vi "Y_N_KeyPress.vi"(8 "error in (no error)":errorcluster) -> (0 "error out":errorcluster, 1 "P/F":bool, 2 "PASS/FAIL":string="FAIL", 3 "Y/N":string="No", 4 "numberKey":i32, 5 "keys pressed":T1(array[ring]))   [LabVIEW 2018]
uses:
  <vilib>/Utility/inputDevices.llb/keyboardAcquire.vi
  <vilib>/Utility/inputDevices.llb/closeKeyboard.vi
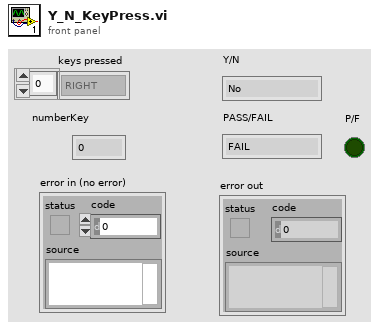
[diagram p1: front panel]
types:
  T1 = enum16{"0", "1", "2", "3", "4", "5", "6", "7", "8", "9", "A", "B", "C", "D", "E", "F", "G", "H", "I", "J", "K", "L", "M", "N", "O", "P", "Q", "R", "S", "T", "U", "V", "W", "X", "Y", "Z", "F1", "F2", "F3", "F4", "F5", "F6", "F7", "F8", "F9", "F10", "F11", "F12", "F13", "F14", "F15", "ADD", "BACK", "BACKSLASH", "CAPITAL", "COMMA", "DECIMAL", "DELETE", "DIVIDE", "DOWN", "END", "EQUALS", "ESCAPE", "GRAVE (`)", "HOME", "INSERT", "LBRACKET", "LCONTROL", "LEFT", "L ALT", "LSHIFT", "LWIN", "MINUS", "MULTIPLY", "NEXT", "NUMLOCK", "NUMPAD_0", "NUMPAD_1", "NUMPAD_2", "NUMPAD_3", "NUMPAD_4", "NUMPAD_5", "NUMPAD_6", "NUMPAD_7", "NUMPAD_8", "NUMPAD_9", "PAUSE", "PERIOD", "PRIOR (PG UP)", "RBRACKET", "RCONTROL", "RETURN", "RIGHT", "R ALT", "RSHIFT", "RWIN", "SCROLL", "SEMICOLON", "SLASH", "SPACE", "SUBTRACT", "TAB", "UP", "ENTER (num pad)", "' (quote)"}[]
  T2 = enum16{"0", "1", "2", "3", "4", "5", "6", "7", "8", "9", "A", "B", "C", "D", "E", "F", "G", "H", "I", "J", "K", "L", "M", "N", "O", "P", "Q", "R", "S", "T", "U", "V", "W", "X", "Y", "Z", "F1", "F2", "F3", "F4", "F5", "F6", "F7", "F8", "F9", "F10", "F11", "F12", "F13", "F14", "F15", "ADD", "BACK", "BACKSLASH", "CAPITAL", "COMMA", "DECIMAL", "DELETE", "DIVIDE", "DOWN", "END", "EQUALS", "ESCAPE", "GRAVE (`)", "HOME", "INSERT", "LBRACKET", "LCONTROL", "LEFT", "L ALT", "LSHIFT", "LWIN", "MINUS", "MULTIPLY", "NEXT", "NUMLOCK", "NUMPAD_0", "NUMPAD_1", "NUMPAD_2", "NUMPAD_3", "NUMPAD_4", "NUMPAD_5", "NUMPAD_6", "NUMPAD_7", "NUMPAD_8", "NUMPAD_9", "PAUSE", "PERIOD", "PRIOR (PG UP)", "RBRACKET", "RCONTROL", "RETURN", "RIGHT", "R ALT", "RSHIFT", "RWIN", "SCROLL", "SEMICOLON", "SLASH", "SPACE", "SUBTRACT", "TAB", "UP", "ENTER (num pad)", "' (quote)"}
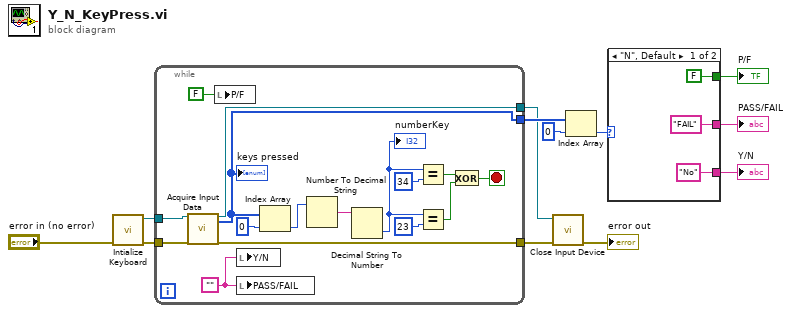
[diagram p0: block diagram]
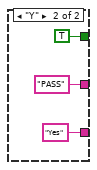
[diagram p2: hidden frame]
diagram:
  n1 = call <vilib>:"Intialize Keyboard.vi"("error in (no error)"="error in (no error)") -> ("error out"=w7:errorcluster, "device ID"=w6:refnum<k1>)  [unwired: 9 in]
  n2 = while {
    tunnel: [w19] -> w12
    tunnel: w7 -> [w18]
    tunnel: w6 -> [w17]
    tunnel: [w16] -> w5
    tunnel: [w15] -> w4
    stop <- w20 stop-if-true
    w14 = ""
    n3 = call-poly <vilib>:"Acquire Input Data.vi"("device ID"=w17, "error in (no error)"=w18) -> ("device ID"=w15:refnum<k1>, "keys pressed"=w19:T1, "error out"=w16:errorcluster)  [unwired: 15 in]
    "keys pressed" <- w19
    n4 = local write "P/F"(FALSE ("Boolean")) -> ()
    n5 = local write "Y/N"(w14) -> ()
    n6 = local write "PASS/FAIL"(w14) -> ()
    n7 = Index Array(array=w19, index=0) -> (element=w27:T2)
    n8 = Number To Decimal String(number=w27) -> (decimal integer string=w26:string)  [unwired: 1 in]
    n9 = Decimal String To Number(string=w26) -> (number=w25:i32)  [unwired: 2 in, 1 out]
    "numberKey" <- w25
    n10 = Equal?(x=w25, y=34) -> (x = y?=w22:bool)
    n11 = Equal?(x=w25, y=23) -> (x = y?=w21:bool)
    n12 = Exclusive Or(1:w21, 2:w22) -> (0:w20:bool)
  }
  n13 = call-poly <vilib>:"Close Input Device.vi"("error in (no error)"=w5, "device ID"=w4) -> ("error out"=→"error out":errorcluster)  [unwired: 8 in]
  n14 = Index Array(array=w12, index=0) -> (element=w10:T2)
  n15 = case shown="\"N\", Default" w10 {
    tunnel: ["No" "Yes"] -> w9
    tunnel: ["FAIL" "PASS"] -> w8
    tunnel: [FALSE TRUE] -> w1
    frame "N", Default {
    }
    frame "Y" {
    }
  }
  "Y/N" <- w9
  "PASS/FAIL" <- w8
  "P/F" <- w1
